vi "Warmup.vi"(7 "FrequencyCounter":refnum<visa-resource-name>, 8 "error in":errorcluster, 9 "connection information":path, 10 "System Number":string, 11 "Arduino in":refnum<visa-resource-name>) -> (0 "error out":errorcluster, 3 "Arduino out":refnum<visa-resource-name>)   [LabVIEW 2024]
uses:
  <vilib>/addons/database/Connection.llb/DB Tools Open Connec (Path).vi
  Agilent 532XX Series/Public/Configure/Measurement/Configure Measurement (Frequency).vi
  <vilib>/Utility/file.llb/Write Delimited Spreadsheet (string).vi
  <vilib>/addons/database/_DB Variant To Data/Database Variant To Data.xnode
  <vilib>/addons/database/NI_Database_API.lvlib
  Agilent 532XX Series/Agilent 532XX Series.lvlib
panel:
  out "StartTime":string
  out "Unit_Number":string
  out "Work Order":string
  out "OscVoltage":string
  out "TimeMeasured":string[](array[string])
  out "Command Array":string[](array[string])
  out "Frequency":string[](array[string])
  out "TimeStart":string
  out "Nominal Frequency":string
  in  "DC_SN":string
  out "IsSine":bool=TRUE
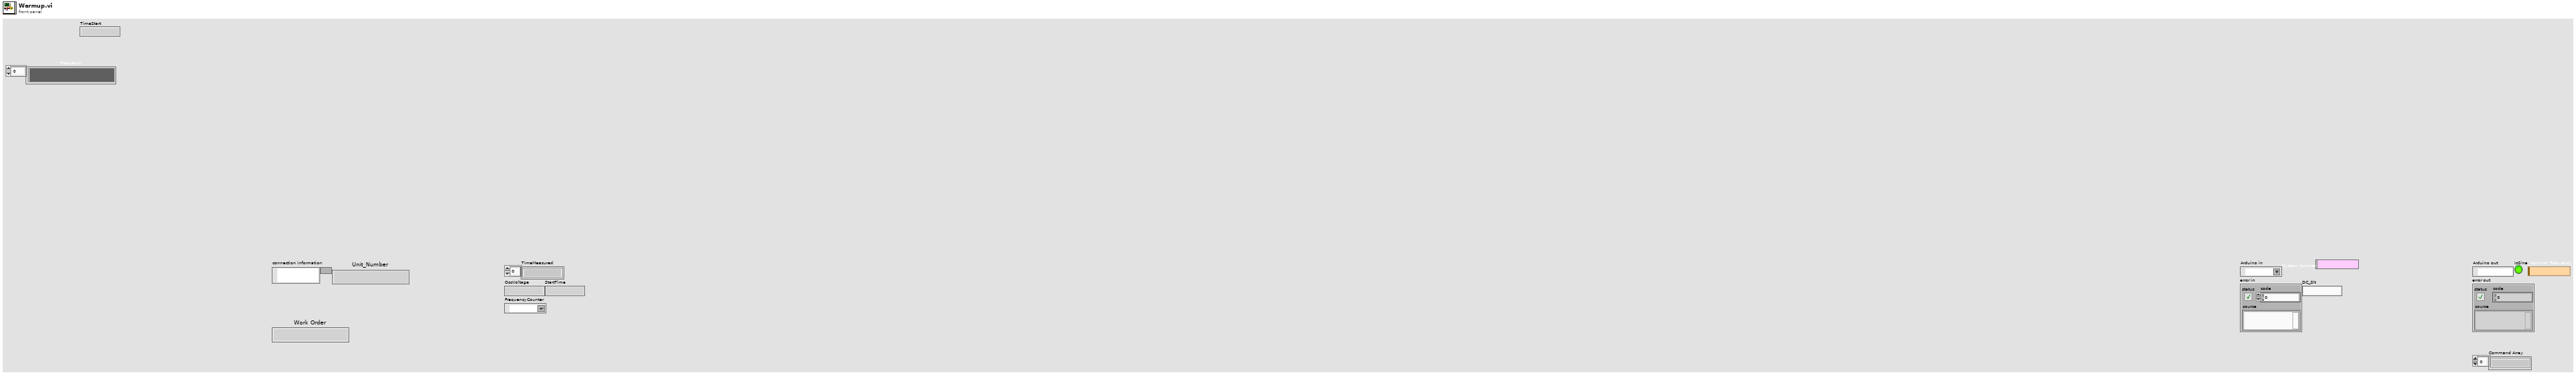
[diagram p1: front panel]
types:
  T1 = typedef "NI_Database_API.lvlib/Conn ObjectReference.ctl" = refnum<k1>
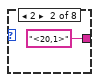
[diagram p3: hidden frame]
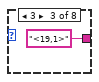
[diagram p4: hidden frame]
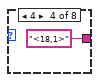
[diagram p5: hidden frame]
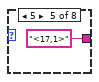
[diagram p6: hidden frame]
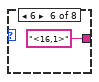
[diagram p7: hidden frame]
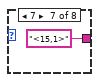
[diagram p8: hidden frame]
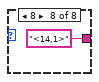
[diagram p9: hidden frame]
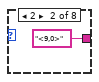
[diagram p10: hidden frame]
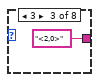
[diagram p11: hidden frame]
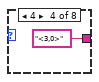
[diagram p12: hidden frame]
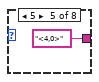
[diagram p13: hidden frame]
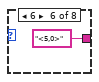
[diagram p14: hidden frame]
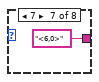
[diagram p15: hidden frame]
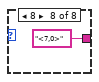
[diagram p16: hidden frame]
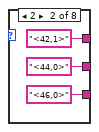
[diagram p17: hidden frame]
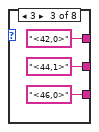
[diagram p18: hidden frame]
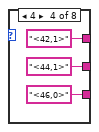
[diagram p19: hidden frame]
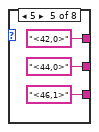
[diagram p20: hidden frame]
diagram:
  n1 = flat-sequence {
    tunnel: [w21] -> w3
    tunnel: [w19] -> w1
    tunnel: [w32] -> w4
    tunnel: w3 -> [w32]
    tunnel: [w31] -> w2
    tunnel: w1 -> [w31]
    tunnel: [w53] -> w7
    tunnel: [w52] -> w5
    tunnel: w4 -> [w50]
    tunnel: w2 -> [w49]
    tunnel: [w64] -> w8
    tunnel: w7 -> [w64]
    tunnel: [w63] -> w6
    tunnel: w5 -> [w63]
    tunnel: [w68] -> w12
    tunnel: [w67] -> w11
    tunnel: w8 -> [w66]
    tunnel: w6 -> [w65]
    tunnel: w12 -> [w755]
    tunnel: w11 -> [w754]
    tunnel: [w755] -> w10
    tunnel: [w754] -> w9
    tunnel: [w759] -> w13
    tunnel: [w760] -> w14
    tunnel: w9 -> [w757]
    tunnel: w10 -> [w758]
    frame #0 {
      n2 = Get Date/Time In Seconds() -> (seconds since 1Jan1904=w29:timestamp)
      n3 = Format Date/Time String(time format string (%c)="%x_%I-%M" ("string"), seconds (now)=w29) -> (date/time string=w28:string)  [unwired: 1 in]
      n4 = Build Array("<48,0>" ("string"), "<50,0>" ("string"), "<52,0>" ("string")) -> (w15:string[])
      n5 = Search and Replace String(replace all?=TRUE ("replace all? (F)"), input string=w28, search string="/", replace string="-" ("replace string (\"\")")) -> (result string=→"StartTime":string)  [unwired: 4 in, 3 out]
      n6 = call "Arduino Command Builder.vi"("error in"="error in", "Commands"=w15, "Arduino in"="Arduino in") -> ("error out"=w19:errorcluster, "Arduino out"=w21:refnum<visa-resource-name>)  [unwired: 7 in]
    }
    frame #1 {
      w37 = 25.0
      n7 = Number To Fractional String(number=w37) -> (F-format string=w36:string)  [unwired: 3 in]
      n8 = Bundle(0, 6) -> (w38:cluster{i32, i32})  [unwired: 1 in]
      n9 = call "Set Temperature and Rise Time.vi"("Slew Time String"="0", "Temperature String"=w36, "Device"=w38) -> ("error out"=w30:errorcluster)  [unwired: 3 in]
      n10 = while {
        tunnel: w38 -> [w42]
        tunnel: w37 -> [w41]
        tunnel: w37 -> [w40]
        tunnel: w30 -> [w39]
        stop <- w48 stop-if-true
        n11 = call "Read Saunders Temperature.vi"("error in"=w39, "Device"=w42) -> ("Temperature"=w47:dbl)  [unwired: 2 in, 1 out]
        n12 = Add(x=0.5, y=w40) -> (x+y=w43:dbl)
        n13 = Subtract(x=w41, y=0.5) -> (x-y=w45:dbl)
        n14 = In Range and Coerce(upper limit=w43, x=w47, lower limit=w45) -> (In Range?=w48:bool)  [unwired: 1 out]
      }
    }
    frame #2 {
      n15 = Build Array("<43,0>" ("y"), "<45,0>" ("y"), "<47,0>" ("y"), "<51,0>" ("y"), "<53,0>" ("y"), "<39,0>" ("y"), "<41,0>" ("y"), "<49,0>" ("y")) -> (w54:string[])
      n16 = call "Arduino Command Builder.vi"("error in"=w49, "Commands"=w54, "Arduino in"=w50) -> ("error out"=w52:errorcluster, "Arduino out"=w53:refnum<visa-resource-name>)  [unwired: 7 in]
    }
    frame #3 {
      n17 = Wait (ms)(milliseconds to wait=u32 300000 ("millisecond multiple")) -> ()  [unwired: 1 out]
    }
    frame #4 {
      n18 = for {
        N: 32 -> [_]
        shift-right: [w71] -> w68
        shift-left: w65 -> [w74]
        shift-right: [w70] -> w67
        shift-left: w66 -> [w73]
        i -> [w72]
        n19 = for {
          N: 8 -> [_]
          shift-right: [w82] -> w71
          shift-left: w74 -> [w87]
          shift-right: [w77] -> w70
          shift-left: w73 -> [w86]
          tunnel: w72 -> [w85]
          i -> [w88]
          n20 = flat-sequence {
            tunnel: w87 -> [w91]
            tunnel: w86 -> [w90]
            tunnel: [w89] -> w81
            tunnel: [w90] -> w78
            tunnel: w88 -> [w114]
            tunnel: w85 -> [w113]
            tunnel: [w112] -> w84
            tunnel: [w111] -> w83
            tunnel: w81 -> [w110]
            tunnel: [w110] -> w80
            tunnel: [w109] -> w79
            tunnel: w78 -> [w109]
            tunnel: [w105] -> w76
            tunnel: w84 -> [w178]
            tunnel: w83 -> [w177]
            tunnel: [w176] -> w82
            tunnel: w80 -> [w175]
            tunnel: w79 -> [w174]
            tunnel: [w173] -> w77
            tunnel: w76 -> [w172]
            frame #0 {
              n21 = call <vilib>:"Clear Errors.vi"("error in (no error)"=w91) -> ("error out"=w89:errorcluster)  [unwired: 5 in, 1 out]
            }
            frame #1 {
              n22 = local write "DC_SN"("" ("DC.SN")) -> ()
              n23 = local read "System Number"() -> (w116:string)
              n24 = local read "connection information"() -> (w92:path)
              n25 = Increment(x=w114) -> (x+1=w112:i32)
              n26 = Number To Decimal String(number=w112) -> (decimal integer string=w117:string)  [unwired: 1 in]
              n27 = Concatenate Strings("WHERE System=" ("SQL Query"), w116, " AND Rack=", w117, ";" ("string")) -> (w93:string)
              n28 = call-poly <vilib>:"DB Tools Open Connection.vi"("connection information"=w92) -> ("error out"=w103:errorcluster, "connection reference"=w104:T1)  [unwired: 7 in]
              n29 = call <vilib>:"DB Tools Select Data.vi"("condition"=w93, "error in (no error)"=w103, "columns"=string[] ["Position"], "table"="ACTIVE", "connection reference"=w104) -> ("error out"=w100:errorcluster, "data"=w98:variant[][], "connection reference out"=w102:T1)  [unwired: 1 in]
              n30 = xnode "Database Variant To Data"("database variant"=w98, "error in (no error)"=w100, "type"=string[][] [] ("DC.SN")) -> ("data"=w97:string[][], "error out"=w101:errorcluster)
              n31 = call <vilib>:"DB Tools Close Connection.vi"("error in (no error)"=w101, "connection reference"=w102) -> ("error out"=w94:errorcluster)  [unwired: 5 in]
              n32 = Index Array(array=w97, index (row)=0 ("disabled index (row)"), index (col)=0 ("disabled index (col)")) -> (element=w127:string)
              n33 = Unbundle By Name(w94) -> ("status"=w108:bool)
              n34 = call <vilib>:"Delimited String to 1D String Array.vi"("delimiter"=",", "delimited string"=w127) -> ("string array"=w124:string[])  [unwired: 9 in]
              n35 = Not(x=w108) -> (.not. x?=w107:bool)
              n36 = Index Array(array=w124, index=w113) -> (element=w123:string)
              n37 = Equal?(x="1", y=w123) -> (x = y?=w106:bool)
              n38 = Increment(x=w113) -> (x+1=w111:i32)
              n39 = And(x=w106, y=w107) -> (x .and. y?=w105:bool)
            }
            frame #2 {
              n40 = case shown="True" w172 {
                tunnel: w178 -> [_ w231]
                tunnel: w177 -> [_ w230]
                tunnel: [w179 w212] -> w176
                tunnel: w175 -> [w179 w227]
                tunnel: w174 -> [w180 w226]
                tunnel: [w180 w214] -> w173
                frame False {
                }
                frame True {
                  n41 = flat-sequence {
                    tunnel: w231 -> [w232]
                    tunnel: w230 -> [w236]
                    tunnel: [w236] -> w229
                    tunnel: [w232] -> w228
                    tunnel: [w235] -> w220
                    tunnel: w228 -> [w466]
                    tunnel: w229 -> [w483]
                    tunnel: [w470] -> w225
                    tunnel: [w469] -> w221
                    tunnel: w220 -> [w469]
                    tunnel: [w466] -> w219
                    tunnel: [w538] -> w213
                    tunnel: w227 -> [w540]
                    tunnel: w226 -> [w541]
                    tunnel: [w539] -> w215
                    tunnel: w225 -> [w537]
                    tunnel: [w537] -> w222
                    tunnel: w221 -> [w536]
                    tunnel: w219 -> [w535]
                    tunnel: [w535] -> w218
                    tunnel: [w550] -> w211
                    tunnel: [w549] -> w210
                    tunnel: w218 -> [w549]
                    tunnel: w222 -> [w550]
                    tunnel: w211 -> [w579]
                    tunnel: [w579] -> w205
                    tunnel: w210 -> [w578]
                    tunnel: [w578] -> w203
                    tunnel: [w568] -> w200
                    tunnel: [w567] -> w198
                    tunnel: w205 -> [w584]
                    tunnel: [w584] -> w204
                    tunnel: w203 -> [w583]
                    tunnel: [w583] -> w202
                    tunnel: [w581] -> w201
                    tunnel: w200 -> [w581]
                    tunnel: [w580] -> w199
                    tunnel: w198 -> [w580]
                    tunnel: w204 -> [w594]
                    tunnel: [w594] -> w207
                    tunnel: w202 -> [w593]
                    tunnel: [w593] -> w206
                    tunnel: w201 -> [w591]
                    tunnel: w199 -> [w587]
                    tunnel: [w596] -> w223
                    tunnel: w207 -> [w596]
                    tunnel: w206 -> [w595]
                    tunnel: [w595] -> w217
                    tunnel: [w602] -> w224
                    tunnel: w223 -> [w602]
                    tunnel: w217 -> [w598]
                    tunnel: [w598] -> w216
                    tunnel: w224 -> [w632]
                    tunnel: w216 -> [w631]
                    tunnel: [w631] -> w185
                    tunnel: w185 -> [w642]
                    tunnel: [w642] -> w184
                    tunnel: [w637] -> w181
                    tunnel: w184 -> [w659]
                    tunnel: [w659] -> w191
                    tunnel: [w644] -> w187
                    tunnel: [w643] -> w182
                    tunnel: w181 -> [w643]
                    tunnel: w191 -> [w678]
                    tunnel: [w678] -> w190
                    tunnel: [w662] -> w188
                    tunnel: w187 -> [w662]
                    tunnel: [w663] -> w186
                    tunnel: [w661] -> w183
                    tunnel: w182 -> [w661]
                    tunnel: w190 -> [w683]
                    tunnel: [w683] -> w189
                    tunnel: w188 -> [w681]
                    tunnel: w186 -> [w680]
                    tunnel: w183 -> [w679]
                    tunnel: w189 -> [w703]
                    tunnel: w215 -> [w708]
                    tunnel: w213 -> [w706]
                    tunnel: [w707] -> w209
                    tunnel: [w705] -> w208
                    tunnel: w209 -> [w735]
                    tunnel: w208 -> [w734]
                    tunnel: [w735] -> w197
                    tunnel: [w734] -> w196
                    tunnel: [w726] -> w192
                    tunnel: w197 -> [w739]
                    tunnel: w196 -> [w738]
                    tunnel: [w739] -> w195
                    tunnel: [w738] -> w194
                    tunnel: [w736] -> w193
                    tunnel: w192 -> [w736]
                    tunnel: [w748] -> w212
                    tunnel: [w749] -> w214
                    tunnel: w195 -> [w749]
                    tunnel: w194 -> [w748]
                    tunnel: w193 -> [w743]
                    frame #0 {
                      n42 = case shown="1, Default" w232 {
                        tunnel: ["<42,0>" ("string") "<42,1>" ("string") "<42,0>" ("string") "<42,1>" ("string") "<42,0>" ("string") "<42,1>" ("string") "<42,0>" ("string") "<42,1>" ("string")] -> w239
                        tunnel: ["<44,0>" ("string") "<44,0>" ("string") "<44,1>" ("string") "<44,1>" ("string") "<44,0>" ("string") "<44,0>" ("string") "<44,1>" ("string") "<44,1>" ("string")] -> w238
                        tunnel: ["<46,0>" ("string") "<46,0>" ("string") "<46,0>" ("string") "<46,0>" ("string") "<46,1>" ("string") "<46,1>" ("string") "<46,1>" ("string") "<46,1>" ("string")] -> w237
                        frame 1, Default {
                        }
                        frame 2 {
                        }
                        frame 3 {
                        }
                        frame 4 {
                        }
                        frame 5 {
                        }
                        frame 6 {
                        }
                        frame 7 {
                        }
                        frame 8 {
                        }
                      }
                      n43 = case shown="1, Default" w232 {
                        tunnel: ["<8,0>" ("string") "<9,0>" ("string") "<2,0>" ("string") "<3,0>" ("string") "<4,0>" ("string") "<5,0>" ("string") "<6,0>" ("string") "<7,0>" ("string")] -> w234
                        frame 1, Default {
                        }
                        frame 2 {
                        }
                        frame 3 {
                        }
                        frame 4 {
                        }
                        frame 5 {
                        }
                        frame 6 {
                        }
                        frame 7 {
                        }
                        frame 8 {
                        }
                      }
                      n44 = case shown="1, Default" w232 {
                        tunnel: ["<21,1>" ("string") "<20,1>" ("string") "<19,1>" ("string") "<18,1>" ("string") "<17,1>" ("string") "<16,1>" ("string") "<15,1>" ("string") "<14,1>" ("string")] -> w233
                        frame 1, Default {
                        }
                        frame 2 {
                        }
                        frame 3 {
                        }
                        frame 4 {
                        }
                        frame 5 {
                        }
                        frame 6 {
                        }
                        frame 7 {
                        }
                        frame 8 {
                        }
                      }
                      n45 = case shown="1, Default" w236 {
                        tunnel: ["<32,0>" ("string") "<32,0>" ("string") "<32,0>" ("string") "<32,0>" ("string") "<32,0>" ("string") "<32,0>" ("string") "<32,0>" ("string") "<32,0>" ("string") "<32,0>" ("string") "<32,0>" ("string") "<32,0>" ("string") "<32,0>" ("string") "<32,0>" ("string") "<32,0>" ("string") "<32,0>" ("string") "<32,0>" ("string") "<32,1>" ("string") "<32,1>" ("string") "<32,1>" ("string") "<32,1>" ("string") "<32,1>" ("string") "<32,1>" ("string") "<32,1>" ("string") "<32,1>" ("string") "<32,1>" ("string") "<32,1>" ("string") "<32,1>" ("string") "<32,1>" ("string") "<32,1>" ("string") "<32,1>" ("string") "<32,1>" ("string") "<32,1>" ("string")] -> w240
                        tunnel: ["<30,0>" ("string") "<30,0>" ("string") "<30,0>" ("string") "<30,0>" ("string") "<30,0>" ("string") "<30,0>" ("string") "<30,0>" ("string") "<30,0>" ("string") "<30,1>" ("string") "<30,1>" ("string") "<30,1>" ("string") "<30,1>" ("string") "<30,1>" ("string") "<30,1>" ("string") "<30,1>" ("string") "<30,1>" ("string") "<30,0>" ("string") "<30,0>" ("string") "<30,0>" ("string") "<30,0>" ("string") "<30,0>" ("string") "<30,0>" ("string") "<30,0>" ("string") "<30,0>" ("string") "<30,1>" ("string") "<30,1>" ("string") "<30,1>" ("string") "<30,1>" ("string") "<30,1>" ("string") "<30,1>" ("string") "<30,1>" ("string") "<30,1>" ("string")] -> w241
                        tunnel: ["<28,0>" ("string") "<28,0>" ("string") "<28,0>" ("string") "<28,0>" ("string") "<28,1>" ("string") "<28,1>" ("string") "<28,1>" ("string") "<28,1>" ("string") "<28,0>" ("string") "<28,0>" ("string") "<28,0>" ("string") "<28,0>" ("string") "<28,1>" ("string") "<28,1>" ("string") "<28,1>" ("string") "<28,1>" ("string") "<28,0>" ("string") "<28,0>" ("string") "<28,0>" ("string") "<28,0>" ("string") "<28,1>" ("string") "<28,1>" ("string") "<28,1>" ("string") "<28,1>" ("string") "<28,0>" ("string") "<28,0>" ("string") "<28,0>" ("string") "<28,0>" ("string") "<28,1>" ("string") "<28,1>" ("string") "<28,1>" ("string") "<28,1>" ("string")] -> w242
                        tunnel: ["<26,0>" ("string") "<26,0>" ("string") "<26,1>" ("string") "<26,1>" ("string") "<26,0>" ("string") "<26,0>" ("string") "<26,1>" ("string") "<26,1>" ("string") "<26,0>" ("string") "<26,0>" ("string") "<26,1>" ("string") "<26,1>" ("string") "<26,0>" ("string") "<26,0>" ("string") "<26,1>" ("string") "<26,1>" ("string") "<26,0>" ("string") "<26,0>" ("string") "<26,1>" ("string") "<26,1>" ("string") "<26,0>" ("string") "<26,0>" ("string") "<26,1>" ("string") "<26,1>" ("string") "<26,0>" ("string") "<26,0>" ("string") "<26,1>" ("string") "<26,1>" ("string") "<26,0>" ("string") "<26,0>" ("string") "<26,1>" ("string") "<26,1>" ("string")] -> w243
                        tunnel: ["<24,0>" ("string") "<24,1>" ("string") "<24,0>" ("string") "<24,1>" ("string") "<24,0>" ("string") "<24,1>" ("string") "<24,0>" ("string") "<24,1>" ("string") "<24,0>" ("string") "<24,1>" ("string") "<24,0>" ("string") "<24,1>" ("string") "<24,0>" ("string") "<24,1>" ("string") "<24,0>" ("string") "<24,1>" ("string") "<24,0>" ("string") "<24,1>" ("string") "<24,0>" ("string") "<24,1>" ("string") "<24,0>" ("string") "<24,1>" ("string") "<24,0>" ("string") "<24,1>" ("string") "<24,0>" ("string") "<24,1>" ("string") "<24,0>" ("string") "<24,1>" ("string") "<24,0>" ("string") "<24,1>" ("string") "<24,0>" ("string") "<24,1>" ("string")] -> w244
                        frame 1, Default {
                        }
                        frame 2 {
                        }
                        frame 3 {
                        }
                        frame 4 {
                        }
                        frame 5 {
                        }
                        frame 6 {
                        }
                        frame 7 {
                        }
                        frame 8 {
                        }
                        frame 9 {
                        }
                        frame 10 {
                        }
                        frame 11 {
                        }
                        frame 12 {
                        }
                        frame 13 {
                        }
                        frame 14 {
                        }
                        frame 15 {
                        }
                        frame 16 {
                        }
                        frame 17 {
                        }
                        frame 18 {
                        }
                        frame 19 {
                        }
                        frame 20 {
                        }
                        frame 21 {
                        }
                        frame 22 {
                        }
                        frame 23 {
                        }
                        frame 24 {
                        }
                        frame 25 {
                        }
                        frame 26 {
                        }
                        frame 27 {
                        }
                        frame 28 {
                        }
                        frame 29 {
                        }
                        frame 30 {
                        }
                        frame 31 {
                        }
                        frame 32 {
                        }
                      }
                      n46 = Build Array(w239, w238, w237, w244, w243, w242, w241, w240, w234, w233) -> (w235:string[])
                    }
                    frame #1 {
                      # "Gets the latest TimeStart from this System/Rack/Position meaning it will be associated with the oscillator that is currently in the spot"
                      n47 = local read "connection information"() -> (w448:path)
                      n48 = local read "System Number"() -> (w490:string)
                      n49 = Number To Decimal String(number=w466) -> (decimal integer string=w488:string)  [unwired: 1 in]
                      n50 = Number To Decimal String(number=w483) -> (decimal integer string=w489:string)  [unwired: 1 in]
                      n51 = Concatenate Strings("WHERE SystemNumber=" ("SQL Query"), w490, "AND RackNumber=" ("string"), w488, "AND PositionNumber=" ("string"), w489, "ORDER BY TimeStart DESC" ("string")) -> (w447:string)
                      n52 = call-poly <vilib>:"DB Tools Open Connection.vi"("connection information"=w448) -> ("error out"=w455:errorcluster, "connection reference"=w456:T1)  [unwired: 7 in]
                      n53 = call <vilib>:"DB Tools Select Data.vi"("condition"=w447, "error in (no error)"=w455, "table"="MASTER", "connection reference"=w456) -> ("error out"=w452:errorcluster, "data"=w450:variant[][], "connection reference out"=w454:T1)  [unwired: 2 in]
                      n54 = xnode "Database Variant To Data"("database variant"=w450, "error in (no error)"=w452, "type"=string[][] [] ("DC.SN")) -> ("data"=w446:string[][], "error out"=w453:errorcluster)
                      n55 = call <vilib>:"DB Tools Close Connection.vi"("error in (no error)"=w453, "connection reference"=w454) -> ("error out"=w445:errorcluster)  [unwired: 5 in]
                      n56 = Index Array(array=w446, index (row)=0 ("disabled index (row)")) -> (element=w462:string[])  [unwired: 1 in]
                      n57 = Unbundle By Name(w445) -> ("status"=w471:bool)
                      n58 = Index Array(array=w462, index=9) -> (element=→"OscVoltage":string)
                      n59 = Index Array(array=w462, index=1) -> (element=w460:string)
                      n60 = Index Array(array=w462, index=2) -> (element=w458:string)
                      n61 = Index Array(array=w462, index=7) -> (element=→"TimeStart":string)
                      n62 = Index Array(array=w462, index=8) -> (element=w479:string)
                      n63 = Index Array(array=w462, index=0) -> (element=w478:string)
                      n64 = Index Array(array=w462, index=12) -> (element=→"Unit_Number":string)
                      n65 = Index Array(array=w462, index=10) -> (element=w480:string)
                      n66 = local write "Nominal Frequency"(w479) -> ()
                      n67 = local write "DC_SN"(w478) -> ()
                      n68 = Concatenate Strings(w460, "-" ("string"), w458) -> (→"Work Order":string)
                      n69 = Equal?(x="Sine", y=w480) -> (x = y?=w481:bool)
                      n70 = local write "IsSine"(w481) -> ()
                      n71 = Not(x=w471) -> (.not. x?=w470:bool)
                    }
                    frame #2 {
                      n72 = case shown="True" w537 {
                        tunnel: w541 -> [w543 w548]
                        tunnel: w540 -> [w542 w547]
                        tunnel: [w543 w546] -> w539
                        tunnel: [w542 w545] -> w538
                        tunnel: w536 -> [_ w544]
                        frame False {
                        }
                        frame True {
                          n73 = call "Arduino Command Builder.vi"("error in"=w547, "Commands"=w544, "Arduino in"=w548) -> ("error out"=w545:errorcluster, "Arduino out"=w546:refnum<visa-resource-name>)  [unwired: 7 in]
                        }
                      }
                    }
                    frame #3 {
                      # "This checks if the wave is sine and changes the settings based on the waveform type"
                      n74 = local read "IsSine"() -> (w551:bool)
                      n75 = case shown="False" w551 {
                        frame False {
                          n76 = flat-sequence {
                            frame #0 {
                              n77 = Send(0:0 ("bus"), 2:i16 3 ("address"), 5:"INP:COUP DC " ("data string")) -> ()  [unwired: 2 in, 3 out]
                            }
                            frame #1 {
                              n78 = Wait (ms)(milliseconds to wait=u32 1000 ("millisecond multiple")) -> ()  [unwired: 1 out]
                            }
                            frame #2 {
                              n79 = Send(0:0 ("bus"), 2:i16 3 ("address"), 5:"INP:IMP 1.0E6" ("data string")) -> ()  [unwired: 2 in, 3 out]
                            }
                          }
                        }
                        frame True {
                          n80 = flat-sequence {
                            frame #0 {
                              n81 = Send(0:0 ("bus"), 2:i16 3 ("address"), 5:"INP:COUP AC " ("data string")) -> ()  [unwired: 2 in, 3 out]
                            }
                            frame #1 {
                              n82 = Wait (ms)(milliseconds to wait=u32 1000 ("millisecond multiple")) -> ()  [unwired: 1 out]
                            }
                            frame #2 {
                              n83 = Send(0:0 ("bus"), 2:i16 3 ("address"), 5:"INP:IMP 50" ("data string")) -> ()  [unwired: 2 in, 3 out]
                            }
                          }
                        }
                      }
                    }
                    frame #4 {
                      w576 = u16 0 items=["channel 1", "channel 2", "channel 3"] ("channel (ch1:0)")
                      # "Sets the current and voltage limits, and ensures they are within a range to prevent anything from blowing up for channel 1"
                      # "Sets the voltage equal to the value of the OscVoltage which is gotten from the part number (channel 1)"
                      n84 = Wait (ms)(milliseconds to wait=u32 1000) -> ()  [unwired: 1 out]
                      n85 = local read "OscVoltage"() -> (w571:string)
                      n86 = Fract/Exp String To Number(string=w571) -> (number=w570:dbl)  [unwired: 3 in, 1 out]
                      n87 = call "Tek PS2520G Configure Supply24.vi"("GPIB #"=u8 0, "voltage limit"=w570, "Address"=u8 8, "channel (ch1:0)"=w576, "current limit"=1.5, "Switch Output"=TRUE, "output (t:on)"=TRUE) -> ("error out"=w567:errorcluster)  [unwired: 1 in]
                      n88 = Divide(x=w570, y=2.0) -> (x/y=w568:dbl)
                    }
                    frame #5 {
                      n89 = Wait (ms)(milliseconds to wait=u32 500 ("millisecond multiple")) -> ()  [unwired: 1 out]
                    }
                    frame #6 {
                      w589 = u16 1 items=["channel 1", "channel 2", "channel 3"] ("channel (ch1:0)")
                      n90 = call "Tek PS2520G Configure Supply24.vi"("GPIB #"=u8 0, "voltage limit"=w591, "Address"=u8 8, "channel (ch1:0)"=w589, "current limit"=1.5, "error in (no error)"=w587, "Switch Output"=TRUE, "output (t:on)"=TRUE) -> ()  [unwired: 1 out]
                    }
                    frame #7 {
                      n91 = Wait (ms)(milliseconds to wait=u32 500 ("millisecond multiple")) -> ()  [unwired: 1 out]
                    }
                    frame #8 {
                      n92 = for {
                        N: 120 -> [_]
                        tunnel: [w605] -> w601 mode=indexing
                        tunnel: [w603] -> w599 mode=indexing
                        n93 = flat-sequence {
                          tunnel: [w624] -> w604
                          tunnel: [w630] -> w605
                          tunnel: w604 -> [w630]
                          tunnel: [w627] -> w603
                          frame #0 {
                            w607 = 1 items=["Channel 1"=1, "Channel 2"=2, "Channel 3"=3] ("Channel (1:Channel 1)")
                            n94 = local read "FrequencyCounter"() -> (w613:refnum<visa-resource-name>)
                            n95 = call "Initialize.vi"("VISA resource name"=w613) -> ("error out"=w618:errorcluster, "VISA resource name out"=w619:refnum<visa-resource-name>)  [unwired: 9 in]
                            n96 = call "Configure Frequency Gate.vi"("error in (no error)"=w618, "Time Resolution (0.1 s)"=0.01 ("number"), "VISA resource name"=w619) -> ("error out"=w609:errorcluster, "VISA resource name out"=w612:refnum<visa-resource-name>)  [unwired: 7 in]
                            n97 = call-poly "Configure Measurement.vi"("error in (no error)"=w609, "Channel (1:Channel 1)"=w607, "VISA resource name"=w612) -> ("error out"=w610:errorcluster, "VISA resource name out"=w611:refnum<visa-resource-name>)  [unwired: 2 in, 5 out]
                            n98 = call "Read Measurement (Single).vi"("error in (no error)"=w610, "VISA resource name"=w611) -> ("error out"=w616:errorcluster, "Measurement"=w615:dbl, "VISA resource name out"=w617:refnum<visa-resource-name>)  [unwired: 7 in]
                            n99 = Not Equal?(x=w615, y=0.0) -> ()  [unwired: 1 out]
                            n100 = call "Close.vi"("error in (no error)"=w616, "VISA resource name"=w617) -> ("error out"=w614:errorcluster)  [unwired: 9 in]
                            n101 = In Range and Coerce(upper limit=5000000000.0, x=w615, lower limit=0.0) -> (coerced(x)=w608:dbl)  [unwired: 1 out]
                            n102 = Unbundle By Name(w614) -> ("status"=w623:bool)
                            n103 = case shown="True" w623 {
                              frame False {
                              }
                              frame True {
                                n104 = local read "FrequencyCounter"() -> (w626:refnum<visa-resource-name>)
                                n105 = VISA Clear(VISA resource name=w626) -> ()  [unwired: 1 in, 2 out]
                              }
                            }
                            n106 = Format Into String(format string="%.6f", w608) -> (resulting string=w624:string)  [unwired: 2 in, 1 out]
                          }
                          frame #1 {
                            n107 = Get Date/Time In Seconds() -> (seconds since 1Jan1904=w629:timestamp)
                            n108 = Format Date/Time String(time format string (%c)="%m/%d/%Y %I:%M:%S%3u %p", seconds (now)=w629) -> (date/time string=w627:string)  [unwired: 1 in]
                          }
                        }
                      }
                      "Frequency" <- w601
                      "TimeMeasured" <- w599
                    }
                    frame #9 {
                      n109 = case shown="True" w632 {
                        frame False {
                        }
                        frame True {
                          n110 = local read "connection information"() -> (w633:path)
                          n111 = local read "TimeMeasured"() -> (w634:string[])
                          n112 = local read "Frequency"() -> (w635:string[])
                          n113 = local read "DC_SN"() -> (w636:string)
                          n114 = call "Warmup Saving.vi"("connection information"=w633, "TimeMeasured"=w634, "DC_SN"=w636, "Frequency"=w635) -> ()  [unwired: 8 in]
                        }
                      }
                    }
                    frame #10 {
                      n115 = local read "TimeMeasured"() -> (w641:string[])
                      n116 = call "TimeToSeconds.vi"("TimesMeasured"=w641) -> ("Seconds Passed"=w640:string[])  [unwired: 10 in]
                      n117 = Insert Into Array(array=w640, index=0, new element="1" ("new element/subarray")) -> (w637:string[])
                    }
                    frame #11 {
                      w652 = "-" ("string")
                      n118 = local read "Unit_Number"() -> (w655:string)
                      n119 = local read "Work Order"() -> (w656:string)
                      n120 = local read "StartTime"() -> (w650:string)
                      n121 = Concatenate Strings("\\\\Bti-dc1\\ate\\Warmup\\" ("string"), "Warmup-" ("string"), w656, w652, w655, w652, w650) -> (w649:string)
                      n122 = local read "DC_SN"() -> (w646:string)
                      n123 = String To Path(string=w649) -> (path=w651:path)
                      n124 = call <vilib>:"Check if File or Folder Exists.vi"("path"=w651) -> ("file or folder exists?"=w658:bool, "dup path"=w657:path)  [unwired: 8 in, 1 out]
                      n125 = Concatenate Strings(w649, "\\" ("string"), w646, ".csv" ("string")) -> (w645:string)
                      n126 = case shown="False" w658 {
                        tunnel: w657 -> [w660 _]
                        frame False {
                          n127 = Create Folder(path (use dialog)=w660) -> ()  [unwired: 2 in, 3 out]
                        }
                        frame True {
                        }
                      }
                      n128 = String To Path(string=w645) -> (path=w644:path)
                    }
                    frame #12 {
                      n129 = Build Array("Part_Number" ("string"), "Serial_Number" ("element"), "Date_Code" ("element"), "Work_Order" ("element"), "System_Number" ("element"), "Fixture_Number" ("element"), "Fixture_Position" ("element"), "Temperature" ("element"), "Frequency" ("element"), "Seconds_Passed" ("element"), "Run_ID" ("element")) -> (w677:string[])
                      n130 = call-poly <vilib>:"Write Delimited Spreadsheet.vi"("file path (dialog if empty)"=w662, "1D data"=w677, "append to file? (new file:F)"=FALSE, "delimiter (\\t)"="," ("delimiter (\\t)")) -> ("error out"=w663:errorcluster)  [unwired: 10 in, 1 out]
                    }
                    frame #13 {
                      n131 = local read "Frequency"() -> (w682:string[])
                      n132 = for {
                        tunnel: w681 -> [w687]
                        tunnel: w680 -> [w686]
                        tunnel: w679 -> [w684] mode=indexing
                        tunnel: w682 -> [w685] mode=indexing
                        n133 = flat-sequence {
                          tunnel: w687 -> [w701]
                          tunnel: w686 -> [w695]
                          tunnel: w685 -> [w692]
                          tunnel: w684 -> [w693]
                          frame #0 {
                            w699 = "" ("element")
                            n134 = local read "System Number"() -> (w690:string)
                            n135 = local read "Unit_Number"() -> (w691:string)
                            n136 = local read "Work Order"() -> (w689:string)
                            n137 = local read "DC_SN"() -> (w688:string)
                            n138 = Build Array(w691, w688, w688, w689, w690, w699, w699, "N/A" ("element"), w692, w693, "1515" ("element")) -> (w696:string[])
                            n139 = call-poly <vilib>:"Write Delimited Spreadsheet.vi"("file path (dialog if empty)"=w701, "1D data"=w696, "append to file? (new file:F)"=TRUE, "error in (no error)"=w695, "delimiter (\\t)"="," ("delimiter (\\t)")) -> ()  [unwired: 9 in, 2 out]
                          }
                        }
                      }
                    }
                    frame #14 {
                      n140 = case shown="1, Default" w703 {
                        tunnel: ["<8,1>" ("string") "<9,1>" ("string") "<2,1>" ("string") "<3,1>" ("string") "<4,1>" ("string") "<5,1>" ("string") "<6,1>" ("string") "<7,1>" ("string")] -> w704
                        frame 1, Default {
                        }
                        frame 2 {
                        }
                        frame 3 {
                        }
                        frame 4 {
                        }
                        frame 5 {
                        }
                        frame 6 {
                        }
                        frame 7 {
                        }
                        frame 8 {
                        }
                      }
                      n141 = case shown="7" w703 {
                        tunnel: ["<21,0>" ("string") "<20,0>" ("string") "<19,0>" ("string") "<18,0>" ("string") "<17,0>" ("string") "<16,0>" ("string") "<15,0>" ("string") "<14,0>" ("string")] -> w702
                        frame 1, Default {
                        }
                        frame 2 {
                        }
                        frame 3 {
                        }
                        frame 4 {
                        }
                        frame 5 {
                        }
                        frame 6 {
                        }
                        frame 7 {
                        }
                        frame 8 {
                        }
                      }
                      n142 = Build Array(w704, w702) -> (w709:string[])
                      n143 = call "Arduino Command Builder.vi"("error in"=w706, "Commands"=w709, "Arduino in"=w708) -> ("error out"=w705:errorcluster, "Arduino out"=w707:refnum<visa-resource-name>)  [unwired: 7 in]
                    }
                    frame #15 {
                      w730 = u16 0 items=["channel 1", "channel 2", "channel 3"] ("channel (ch1:0)")
                      n144 = call "Tek PS2520G Configure Supply24.vi"("GPIB #"=u8 0, "voltage limit"=0.0, "Address"=u8 8, "channel (ch1:0)"=w730, "current limit"=1.5, "Switch Output"=FALSE, "output (t:on)"=FALSE) -> ("error out"=w726:errorcluster)  [unwired: 1 in]
                    }
                    frame #16 {
                      n145 = Wait (ms)(milliseconds to wait=u32 500 ("millisecond multiple")) -> ()  [unwired: 1 out]
                    }
                    frame #17 {
                      w740 = u16 1 items=["channel 1", "channel 2", "channel 3"] ("channel (ch1:0)")
                      n146 = call "Tek PS2520G Configure Supply24.vi"("GPIB #"=u8 0, "voltage limit"=0.0, "Address"=u8 8, "channel (ch1:0)"=w740, "current limit"=1.5, "error in (no error)"=w743, "Switch Output"=FALSE, "output (t:on)"=FALSE) -> ()  [unwired: 1 out]
                    }
                  }
                }
              }
            }
          }
        }
      }
    }
    frame #5 {
      # "Turns off Saunders Temp Machine"
      n147 = Bundle(0, 6) -> (w753:cluster{i32, i32})  [unwired: 1 in]
      n148 = call "Set Temperature and Rise Time.vi"("Temperature String"="o", "Device"=w753) -> ()  [unwired: 4 in, 1 out]
    }
    frame #6 {
      n149 = local read "System Number"() -> (w756:string)
      n150 = call "Databse State Checker Testing.vi"("error in"=w758, "System Number"=w756, "Arduino"=w757) -> ("error out"=w760:errorcluster, "Arduino out"=w759:refnum<visa-resource-name>)  [unwired: 7 in]
    }
  }
  "Arduino out" <- w13
  "error out" <- w14
